vi "Get PyObject and Method Names.vi"(8 "error in (no error)":errorcluster, 11 "Call in":refnum<class "Call.lvclass">) -> (0 "error out":errorcluster, 1 "Method Name":string, 2 "PyObject Name":string, 3 "Call out":refnum<class "Call.lvclass">, 4 "Arguments String":string)   [LabVIEW 2020, in "jki_python_bridge.lvlib" / "Call.lvclass"]
uses:
  Call.lvclass
  Call.lvclass/Call.ctl
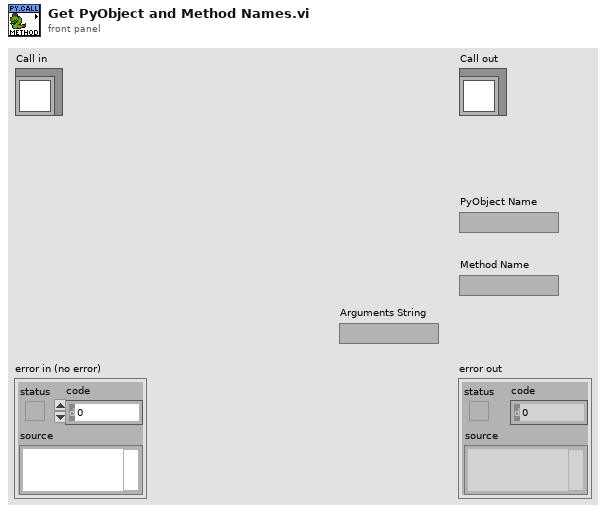
[diagram p1: front panel]
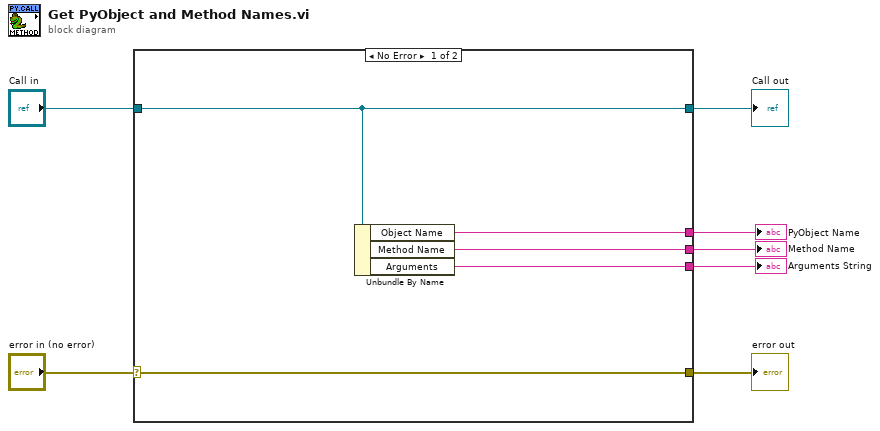
[diagram p0: block diagram]
diagram:
  n1 = case shown="No Error" "error in (no error)" {
    selector: "error in (no error)" -> [w12 w14]
    tunnel: [w12 w14] -> w6
    tunnel: [w11 w13] -> w4
    tunnel: "Call in" -> [w11 w13]
    tunnel: [w10 _] -> w3
    tunnel: [w9 _] -> w2
    tunnel: [w8 _] -> w1
    frame No Error {
      n2 = Unbundle By Name(w11) -> ("Object Name"=w9:string, "Method Name"=w10:string, "Arguments"=w8:string)
    }
    frame Error {
    }
  }
  "error out" <- w6
  "Call out" <- w4
  "Method Name" <- w3
  "PyObject Name" <- w2
  "Arguments String" <- w1
